vi "Example_FPGA_O2_revd.vi"() -> ()   [LabVIEW 2011]
uses:
  <vilib>/Platform/TimedLoop/XDataNode/timing_clust.ctl
  <vilib>/Platform/TimedLoop/XDataNode/nitl_modes.ctl
  <vilib>/Platform/TimedLoop/XDataNode/wakeup.ctl
  <vilib>/Platform/TimedLoop/XDataNode/XDataNode.xnode
  <vilib>/Platform/TimedLoop/XDataNode/XDNodeRunTimeDep.lvlib
panel:
  out "UEGOData":T1
  in  "UEGOControl":T2={"ModuleEnable"=FALSE, "WatchdogIn"=FALSE, "UEGO1Hot"=FALSE, "UEGO2Hot"=FALSE, "Cal1Request"=FALSE, "Cal2Request"=FALSE, "UEGOHeaterPeriod"=17857, "UEGO1HeaterPulseWidth"=0, "UEGO2HeaterPulseWidth"=0}
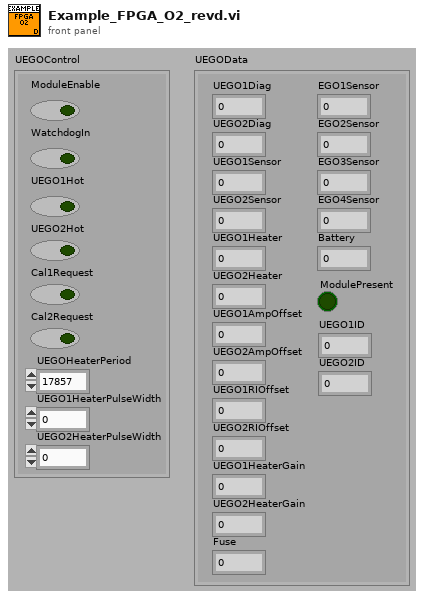
[diagram p1: front panel]
types:
  T1 = cluster{"UEGO1Diag":u8, "UEGO2Diag":u8, "UEGO1Sensor":i16, "UEGO2Sensor":i16, "UEGO1Heater":i16, "UEGO2Heater":i16, "UEGO1AmpOffset":i16, "UEGO2AmpOffset":i16, "UEGO1RIOffset":i16, "UEGO2RIOffset":i16, "UEGO1HeaterGain":i16, "UEGO2HeaterGain":i16, "Fuse":i16, "EGO1Sensor":i16, "EGO2Sensor":i16, "EGO3Sensor":i16, "EGO4Sensor":i16, "Battery":i16, "ModulePresent":bool, "UEGO1ID":u8, "UEGO2ID":u8}
  T2 = cluster{"ModuleEnable":bool, "WatchdogIn":bool, "UEGO1Hot":bool, "UEGO2Hot":bool, "Cal1Request":bool, "Cal2Request":bool, "UEGOHeaterPeriod":u16, "UEGO1HeaterPulseWidth":u16, "UEGO2HeaterPulseWidth":u16}
  T3 = typedef "XDNodeRunTimeDep.lvlib/timing_clust.ctl" = cluster{"Expected End [f-1]":u64, "Actual End [f-1]":u64, "Finished Late? [f-1]":bool, "Expected End [i-1]":u64, "Actual End [i-1]":u64, "Finished Late? [i-1]":bool, "Expected Start [i]":u64, "Actual Start [i]":u64, "Expected Start [f]":u64, "Actual Start [f]":u64, "Source Name":string, "Structure Name":string, "Period":i64, "Deadline":i64, "Offset":i64, "Start":i64, "Priority":i32, "Timeout":i32, "Mode":T4, "Wakeup Reason":T5, "Error":errorcluster, "Source Type":string, "Secondary Source Type":string, "Global End Time":u64, "Global Start Time":u64, "Frame Duration":u64, "Iteration Duration":u64, "Assigned CPU":i32, "I/O Scan Engine Mode":u32}
  T4 = typedef "XDNodeRunTimeDep.lvlib/nitl_modes.ctl" = enum32{"No Change", "Process missed periods, maintain original phase", "Discard missed periods, maintain original phase", "Process missed periods, ignore original phase", "Discard missed periods, ignore original phase"}
  T5 = typedef "XDNodeRunTimeDep.lvlib/wakeup.ctl" = enum32{"Normal", "Aborted", "Asynchronous wakeup", "Timing source error", "Timed loop error", "Timeout"}
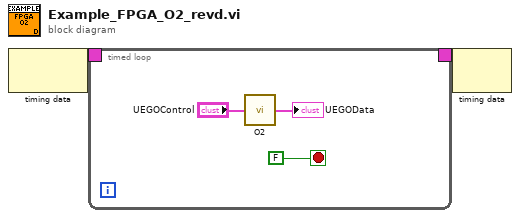
[diagram p0: block diagram]
diagram:
  n1 = node-c288() -> (w1:T3)  [unwired: 1 out]
  n2 = timed-loop {
    timing-out: [_] -> w2
    timing: w1 -> [_]
    stop <- FALSE stop-if-true
    n3 = call "O2"("O2_Control"="UEGOControl") -> ("O2_Data"=→"UEGOData":T1)
  }
  n4 = node-c288(w2) -> ()  [unwired: 1 out]
